vi "Set Render Draw Colour.vi"(6 "B":u8, 7 "A":u8, 8 "error in (no error)":errorcluster, 9 "G":u8, 10 "R":u8, 11 "Renderer Pointer":u32 format="%.0x") -> (0 "error out":errorcluster, 3 "Return":i32)   [LabVIEW 2015, in "LibSDL2.lvlib"]
doc: "Uses the surface to determine the correct pixel format."
uses:
  LibSDL2.lvlib
  DLL/SDL2.dll
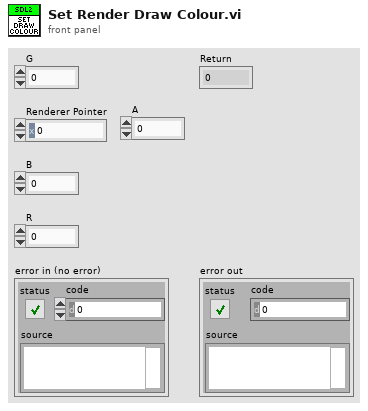
[diagram p1: front panel]
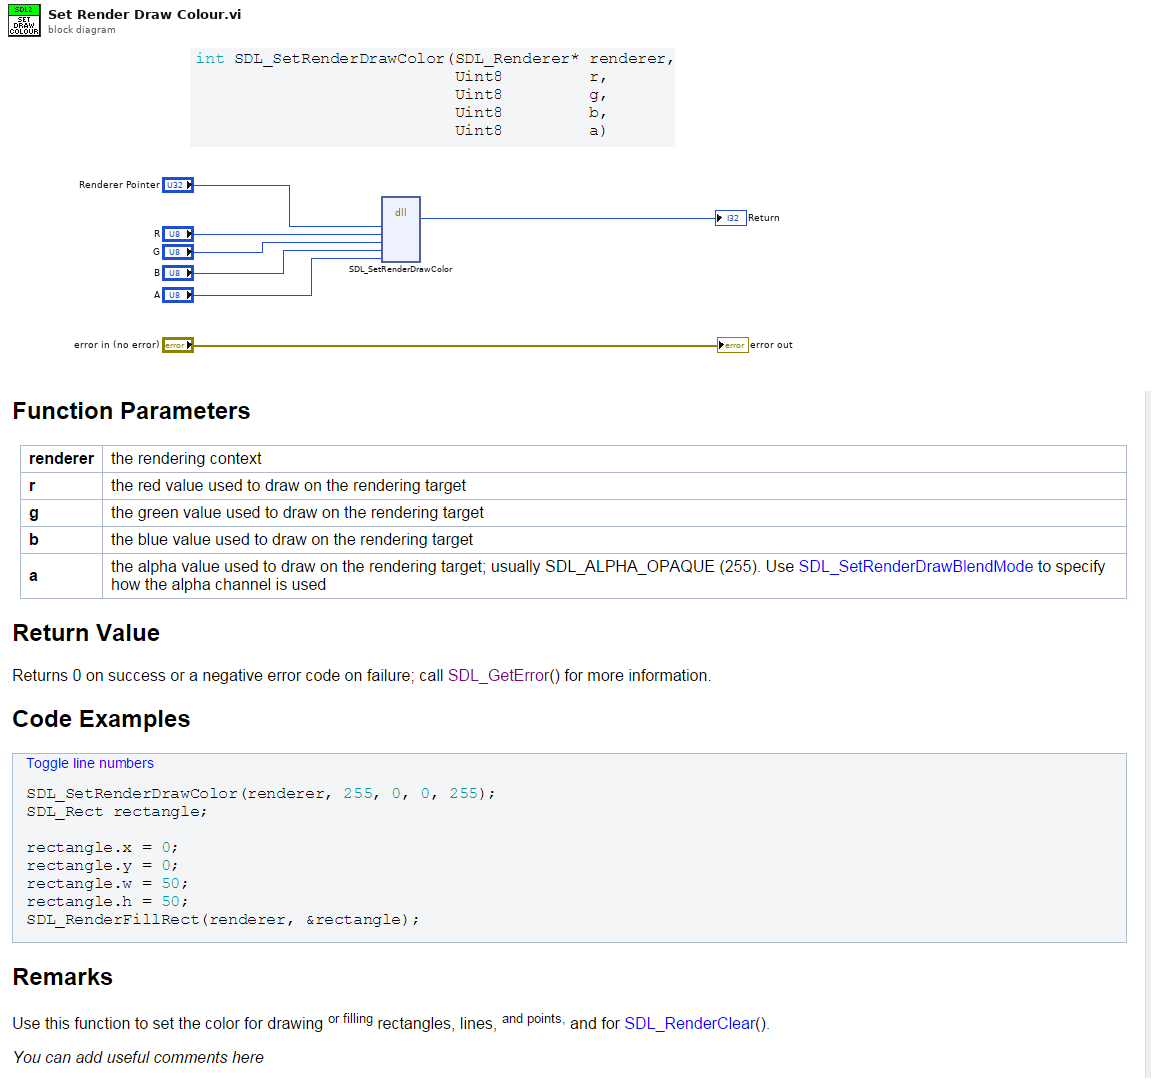
[diagram p0: block diagram]
diagram:
  n1 = dll-call lib="C:/dev/PGS/LabSDL2/Source/Libraries/LibSDL2 Wrapper/DLL/SDL2.dll" fn="SDL_SetRenderDrawColor"("renderer_pointer"="Renderer Pointer", "r"="R", "g"="G", "b"="B", "a"="A") -> ("return type"=→"Return":i32)  [unwired: 8 in, 2 out]
  "error out" <- "error in (no error)"
